vi "Lidar Wrapper (SubVI).vi"(11 "VISA Refnum in":refnum<visa-resource-name>) -> (1 "Array":dbl[](array[numeric]), 2 "Distance Array":u32[](array[numeric]), 3 "VISA Refnum out":refnum<visa-resource-name>)   [LabVIEW 2017]
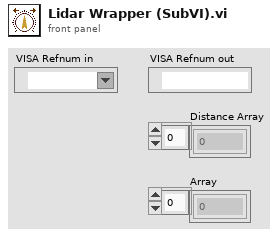
[diagram p1: front panel]
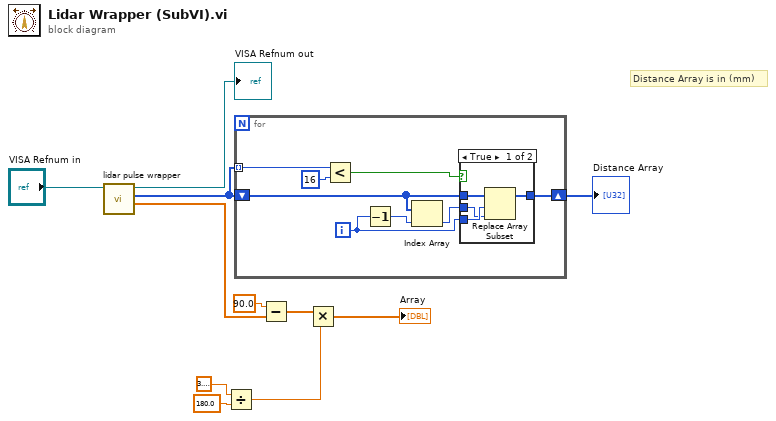
[diagram p0: block diagram]
diagram:
  # "Distance Array is in (mm)"
  n1 = call "lidar pulse wrapper.vi"("VISA resource name"="VISA Refnum in") -> ("Angle Array"=w8:dbl[], "Distance Array"=w10:u32[], "VISA resource name out"=→"VISA Refnum out":refnum<visa-resource-name>)  [unwired: 8 in]
  n2 = Divide(x=3.141592653589793, y=180.0) -> (x/y=w2:dbl)
  n3 = for {
    tunnel: w10 -> [w19] mode=indexing
    shift-right: [w12] -> w11
    shift-left: w10 -> [w14]
    i -> [w16]
    n4 = Less?(x=w19, y=u32 16) -> (x < y?=w17:bool)
    n5 = Decrement(x=w16) -> (x-1=w15:i32)
    n6 = Index Array(array=w14, index=w15) -> (element=w13:u32)
    n7 = case shown="True" w17 {
      tunnel: w16 -> [w23 _]
      tunnel: [w20 w24] -> w12
      tunnel: w14 -> [w22 w24]
      tunnel: w13 -> [w21 _]
      frame True {
        n8 = Replace Array Subset(array=w22, new element=w21, index=w23) -> (w20:u32[])
      }
      frame False {
      }
    }
  }
  "Distance Array" <- w11
  n9 = Subtract(x=90.0 ("y"), y=w8) -> (x-y=w5:dbl[])
  n10 = Multiply(x=w5, y=w2) -> (x*y=→"Array":dbl[])
